vi "Match Template.vi"() -> ()   [LabVIEW 2018]
doc: "Match Template: This example is a template matching example that can be used to find the most similar part to a predefined template in an image."
uses:
  vi.lib/VIRobotics/opencv_yiku/Mat/Mat_8U/Mat_8U.lvclass
  D:/Program Files/company/National Instruments/LabVIEW 2018/vi.lib/addons/VIRobotics/opencv_yiku/Mat/Mat/Mat.lvclass
  vi.lib/VIRobotics/opencv_yiku/Mat/Create_Mat_8U.vi
  vi.lib/VIRobotics/opencv_yiku/opencv_yiku.lvlib
  vi.lib/VIRobotics/opencv_yiku/Mat/Mat/Mat.lvclass
panel:
  out "x-y":dbl[](array[numeric])
  out "Waveform Graph":dbl[][](graph)
  out "new picture":picture
  # "Overview: Demonstrates how to search for an object in an image using Template Matching.\nRequirements: Windows.\nInstructions: \n1.Run the VI."
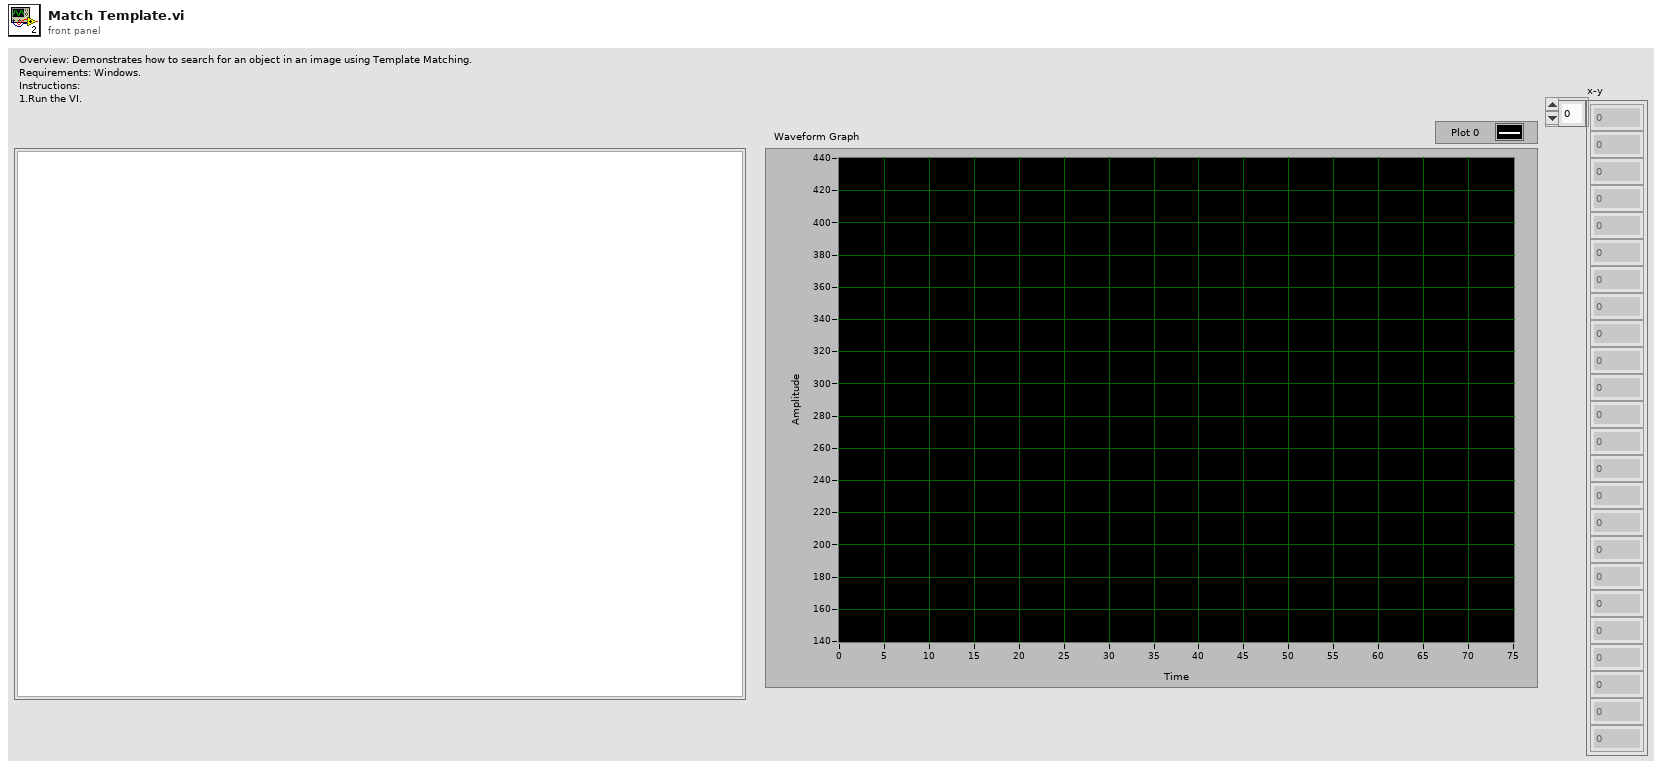
[diagram p1: front panel]
types:
  T1 = enum32{"COLOR_BGR2BGRA", "COLOR_BGRA2BGR", "COLOR_BGR2RGBA", "COLOR_RGBA2BGR", "COLOR_BGR2RGB", "COLOR_BGRA2RGBA", "COLOR_BGR2GRAY", "COLOR_RGB2GRAY", "COLOR_GRAY2BGR", "COLOR_GRAY2BGRA"}
  T2 = cluster{"Width":u16, "Style":enum32{"Solid", "Dash", "Dot", "DashDot", "DashDotDot"}}
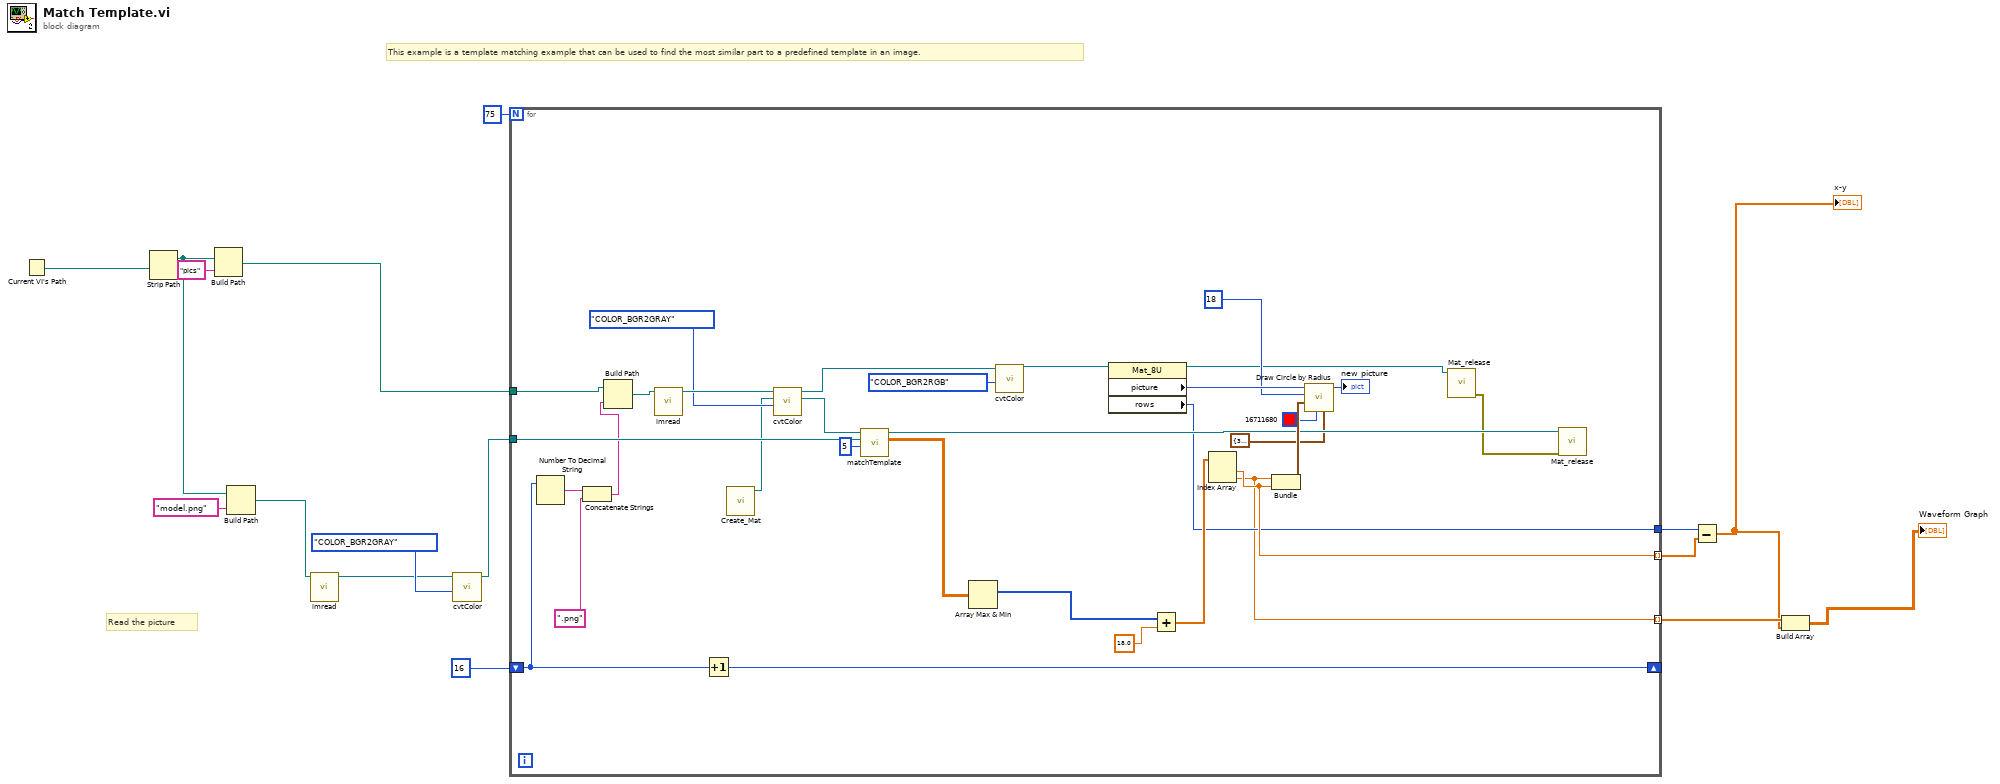
[diagram p0: block diagram]
diagram:
  # "This example is a template matching example that can be used to find the most similar part to a predefined template in an image."
  # "Read the picture"
  n1 = Current VI's Path() -> (path=w6:path)
  n2 = Strip Path(path=w6) -> (stripped path=w2:path)  [unwired: 1 out]
  n3 = Build Path(base path=w2, name or relative path="pics") -> (appended path=w4:path)
  n4 = Build Path(base path=w2, name or relative path="model.png") -> (appended path=w1:path)
  n5 = call "imread.vi"("path"=w1) -> ("Mat out"=w15:refnum<class "Mat_8U.lvclass">)  [unwired: 9 in, 1 out]
  n6 = call "cvtColor.vi"("dstCn"=T1."COLOR_BGR2GRAY", "src"=w15) -> ("src out"=w14:refnum<class "Mat_8U.lvclass">)  [unwired: 7 in, 2 out]
  n7 = for {
    N: 75 -> [_]
    tunnel: w4 -> [w23]
    tunnel: w14 -> [w45]
    shift-right: [w27] -> _
    shift-left: 16 -> [w26]
    tunnel: [w20] -> w11 mode=indexing
    tunnel: [w19] -> w10
    tunnel: [w18] -> w9 mode=indexing
    n8 = Number To Decimal String(number=w26) -> (decimal integer string=w25:string)  [unwired: 1 in]
    n9 = Concatenate Strings(w25, ".png" ("string")) -> (w22:string)
    n10 = Build Path(base path=w23, name or relative path=w22) -> (appended path=w21:path)
    n11 = call "imread.vi"("path"=w21) -> ("Mat out"=w48:refnum<class "Mat_8U.lvclass">)  [unwired: 9 in, 1 out]
    n12 = Increment(x=w26) -> (x+1=w27:i32)
    n13 = call-poly "Create_Mat.vi"() -> ("Mat_8U_out"=w17:refnum<class "Mat_8U.lvclass">)  [unwired: 10 in, 1 out]
    n14 = call "cvtColor.vi"("dstCn"=T1."COLOR_BGR2GRAY", "dst"=w17, "src"=w48) -> ("dst out"=w46:refnum<class "Mat_8U.lvclass">, "src out"=w42:refnum<class "Mat_8U.lvclass">)  [unwired: 6 in, 1 out]
    n15 = call "matchTemplate.vi"("method"=5, "templ"=w45, "src"=w46) -> ("2d_data"=w43:sgl[][], "src out"=w32:refnum<class "Mat_8U.lvclass">)  [unwired: 6 in, 1 out]
    n16 = Array Max & Min(array=w43) -> (max index (indices)=w36:i32[])  [unwired: 3 out]
    n17 = call "cvtColor.vi"("dstCn"=T1."COLOR_BGR2RGB", "src"=w42) -> ("src out"=w40:refnum<class "Mat_8U.lvclass">)  [unwired: 7 in, 2 out]
    n18 = property class="Mat_8U"(reference=w40) -> (reference out=w31:refnum<class "Mat_8U.lvclass">, "picture"=w38:picture, "rows"=w19:i32)  [unwired: 1 in, 1 out]
    n19 = Add(x=w36, y=18.0) -> (x+y=w35:dbl[])
    n20 = Index Array(array=w35) -> (element #1=w20:dbl, element #2=w18:dbl)  [unwired: 2 in]
    n21 = Bundle(w18, w20) -> (w34:cluster{dbl, dbl})  [unwired: 1 in]
    n22 = call <vilib>:"Draw Circle by Radius.vi"("pen"=T2 {"Width"=3, "Style"=enum."Solid"}, "color(black)"=u32 16711680, "pixel center"=w34, "radius"=i16 18, "picture"=w38) -> ("new picture"=→"new picture":picture)  [unwired: 6 in]
    n23 = call "Mat_release.vi"("Mat in"=w31) -> ("error out"=w30:errorcluster)  [unwired: 10 in]
    n24 = call "Mat_release.vi"("error in (no error)"=w30, "Mat in"=w32) -> ()  [unwired: 9 in, 1 out]
  }
  n25 = Subtract(x=w10, y=w11) -> (x-y=w8:dbl[])
  "x-y" <- w8
  n26 = Build Array(w9, w8) -> (→"Waveform Graph":dbl[][])
